vi "onetest.vi"(7 "N":dbl=100000.0) -> ()   [LabVIEW 2016]
panel:
  out "XY Graph":cluster{i32[], dbl[]}(graph)
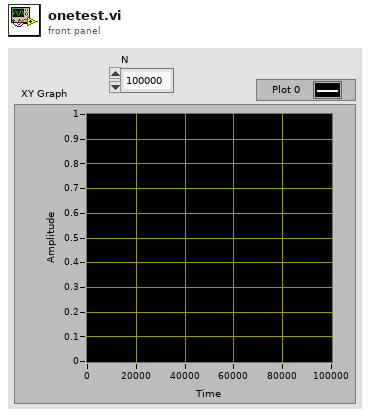
[diagram p1: front panel]
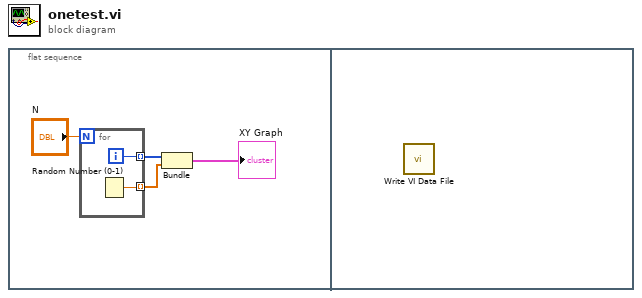
[diagram p0: block diagram]
diagram:
  n1 = flat-sequence {
    frame #0 {
      n2 = for {
        N: "N" -> [_]
        tunnel: [w6] -> w3 mode=indexing
        tunnel: [w5] -> w4 mode=indexing
        i -> [w5]
        n3 = Random Number (0-1)() -> (number: 0 to 1=w6:dbl)
      }
      n4 = Bundle(w4, w3) -> (→"XY Graph":cluster{i32[], dbl[]})  [unwired: 1 in]
    }
    frame #1 {
      n5 = call "Write VI Data File.vi"() -> ()  [unwired: 10 in, 2 out]
    }
  }
